vi "Indruder_UltraSonic+Touch.vi"() -> ()   [LabVIEW 2020]
uses:
  <vilib>/httpClient/LabVIEWHTTPClient.lvlib
  <vilib>/Instr/_visa.llb/VISA Configure Serial Port (Instr).vi
  <vilib>/Instr/_visa.llb/VISA Flush IO Buffer Mask.ctl
panel:
  out "output 2":dbl
  out "output 1":i32
  out "Centimeters":i32
  out "Error Out":errorcluster
  in  "System Armed?":bool
  out "Boolean":bool
  out "Iteration":i32
  out "Present (s)":dbl
  out "Elapsed Time (s)":dbl
  in  "STOP":bool
  out "INTRUDER ALERT!":bool
  in  "Simulated PIR Sensor":bool
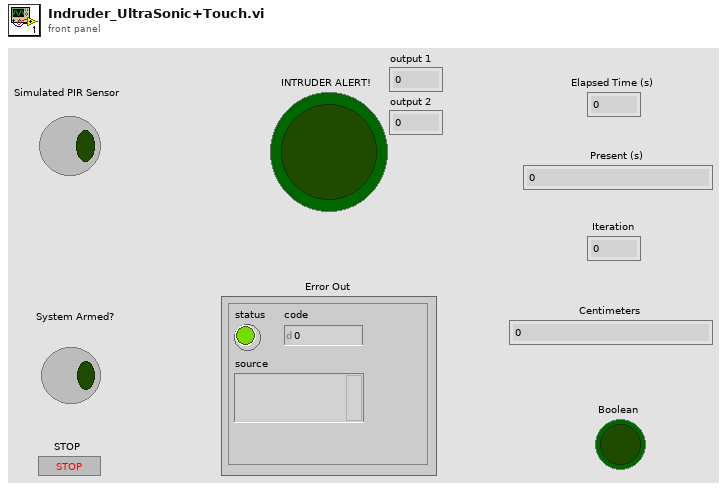
[diagram p1: front panel]
types:
  T1 = typedef "VISA Flush IO Buffer Mask.ctl" = u16
  T2 = typedef "LabVIEWHTTPClient.lvlib/ClientHandle.ctl" = refnum<k1>
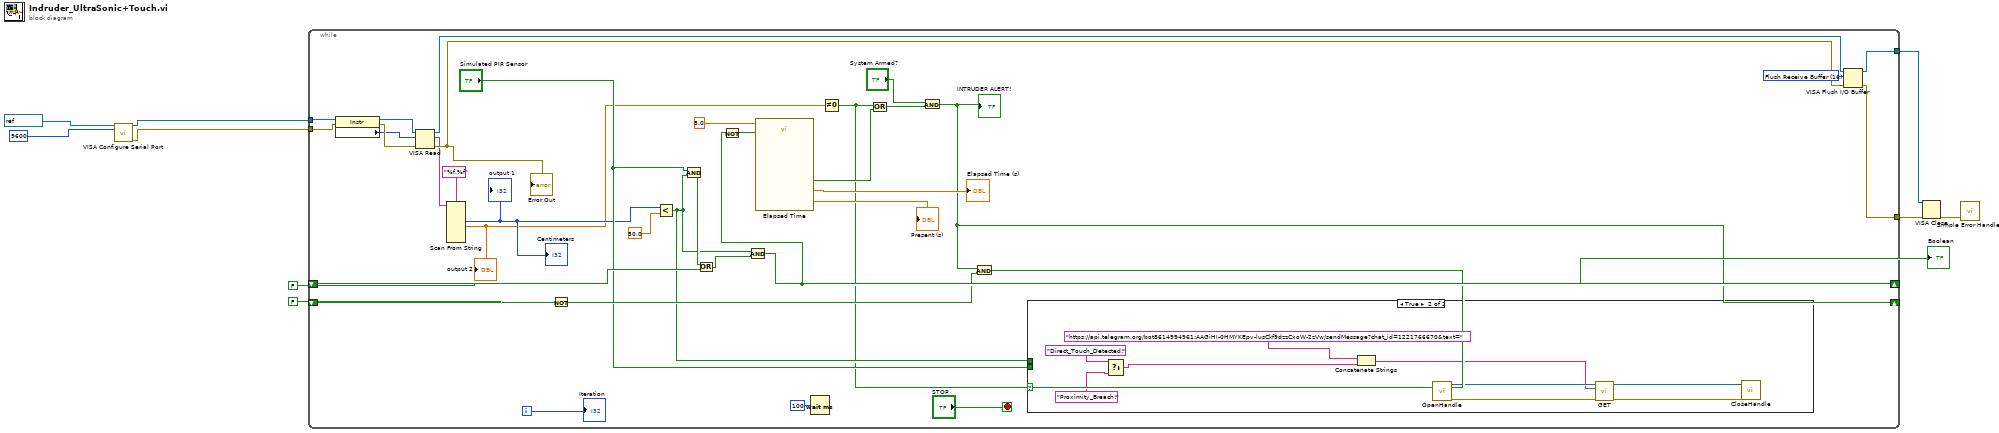
[diagram p0: block diagram]
diagram:
  n1 = call-poly "VISA Configure Serial Port"("VISA resource name"=refnum<visa-resource-name> "COM4", "baud rate (9600)"=u32 9600) -> ("VISA resource name out"=w5:refnum<visa-resource-name>, "error out"=w4:errorcluster)  [unwired: 12 in]
  n2 = while {
    shift-right: [w40] -> w9
    shift-left: FALSE -> [w39]
    shift-right: [w29] -> _
    shift-left: FALSE -> [w31]
    tunnel: w5 -> [w26]
    tunnel: w4 -> [w25]
    tunnel: [w21] -> w2
    tunnel: [w20] -> w1
    i -> [w35]
    stop <- "STOP" stop-if-true
    w17 = T1 16 items=["Flush Receive Buffer"=16, "Write Transmit Buffer to Device"=32, "Flush Receive Buffer (No I/O)"=64, "Flush Transmit Buffer"=128] ("Mask")
    n3 = property class="Instr"(reference=w26, error in=w25) -> (reference out=w24:refnum<visa-resource-name>, error out=w23:errorcluster, "Serial Settings:Number of Bytes at Serial Port"=w22:u32)
    n4 = VISA Read(VISA resource name=w24, byte count=w22, error in (no error)=w23) -> (VISA resource name out=w19:refnum<visa-resource-name>, read buffer=w15:string, error out=w18:errorcluster)  [unwired: 1 out]
    "Error Out" <- w18
    n5 = Scan From String(format string="%f,%f", input string=w15) -> (output 1=w13:i32, output 2=w12:dbl)  [unwired: 10 in, 3 out]
    "Centimeters" <- w13
    "output 1" <- w13
    "output 2" <- w12
    n6 = Not(x=w31) -> (.not. x?=w30:bool)
    n7 = Less?(x=w13, y=50.0) -> (x < y?=w27:bool)
    n8 = And(x="Simulated PIR Sensor", y=w27) -> (x .and. y?=w42:bool)
    n9 = Or(x=w42, y=w39) -> (x .or. y?=w44:bool)
    n10 = And(x=w27, y=w44) -> (x .and. y?=w40:bool)
    n11 = Not(x=w40) -> (.not. x?=w34:bool)
    n12 = call "Elapsed Time"("Time Target (s)"=5.0, "Reset"=w34) -> ("Present (s)"=→"Present (s)":dbl, "Elapsed Time (s)"=→"Elapsed Time (s)":dbl, "Time has Elapsed"=w41:bool)  [unwired: 10 in, 5 out]
    n13 = Wait (ms)(milliseconds to wait=u32 100) -> ()  [unwired: 1 out]
    n14 = Not Equal To 0?(x=w12) -> (x != 0?=w11:bool)
    n15 = Or(x=w11, y=w41) -> (x .or. y?=w33:bool)
    n16 = And(x="System Armed?", y=w33) -> (x .and. y?=w29:bool)
    "INTRUDER ALERT!" <- w29
    n17 = And(x=w29, y=w30, x .and. y?=w11) -> ()
    n18 = case shown="True" w11 {
      tunnel: "Simulated PIR Sensor" -> [_ _]
      tunnel: w27 -> [_ _]
      frame False {
      }
      frame True {
        n19 = Select(t="Direct_Touch_Detected!", f="Proximity_Breach!") -> (s? t:f=w49:string)  [unwired: 1 in]
        n20 = Concatenate Strings("https://api.telegram.org/bot8614994961:AAGiHI-0HMYKEpv-lusCkf9dzzCxoW-2zVw/sendMessage?chat_id=1221766670&text=", w49) -> (w46:string)
        n21 = call <vilib>:"OpenHandle.vi"() -> ("client handle out"=w54:T2, "error out"=w53:errorcluster)  [unwired: 14 in]
        n22 = call <vilib>:"GET.vi"("client handle"=w54, "url"=w46, "error in (no error)"=w53) -> ("client handle out"=w52:T2, "error out"=w51:errorcluster)  [unwired: 9 in, 2 out]
        n23 = call <vilib>:"CloseHandle.vi"("client handle"=w52, "error in (no error)"=w51) -> ()  [unwired: 13 in, 1 out]
      }
    }
    n24 = VISA Flush I/O Buffer(VISA resource name=w19, mask (16)=w17, error in (no error)=w18) -> (VISA resource name out=w21:refnum<visa-resource-name>, error out=w20:errorcluster)
    "Iteration" <- w35
  }
  "Boolean" <- w9
  n25 = VISA Close(VISA resource name=w2, error in (no error)=w1) -> (error out=w3:errorcluster)
  n26 = call <vilib>:"Simple Error Handler.vi"("error in (no error)"=w3) -> ()  [unwired: 4 in, 5 out]
